vi "D2A_5V.vi"(0 "Channel to Cal":T2, 11 "Data In":dbl format="%0.2f", 13 "Cal Unit":T1) -> (15 "Data Out":dbl)   [LabVIEW 2019]
uses:
  Type Defs/New Channel Type Def (RIO).ctl
  Type Defs/Units Type Def (DAQ Rack).ctl
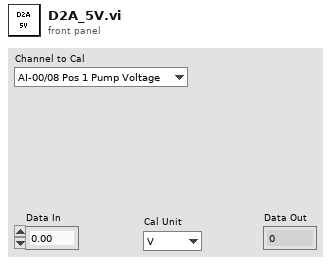
[diagram p1: front panel]
types:
  T1 = typedef "Units Type Def (DAQ Rack).ctl" = enum16{"V", "mA", "A", "Hz", "deg C"}
  T2 = typedef "New Channel Type Def (RIO).ctl" = enum16{"AI-00/08 Pos 1 Pump Voltage", "AI-01/09 Pos 2 Pump Voltage", "AI-02/10 Pos 3 Pump Voltage", "AI-03/11 Pos 4 Pump Voltage", "AI-04/12 Pos 5 Pump Voltage", "AI-05/13 Pos 6 Pump Voltage", "AI-06 Spare", "AI-14 Spare", "AI-07 Spare", "AI-15 Power Supply Voltage", "AI-16 Pos 1 Pump Current", "AI-17 Pos 2 Pump Current", "AI-18 Pos 3 Pump Current", "AI-19 Pos 4 Pump Current", "AI-20 Pos 5 Pump Current", "AI-21 Pos 6 Pump Current", "AI-16 Pos 1 Pump Speed", "AI-17 Pos 2 Pump Speed", "AI-18 Pos 3 Pump Speed", "AI-19 Pos 4 Pump Speed", "AI-20 Pos 5 Pump Speed", "AI-21 Pos 6 Pump Speed", "AI-22 Pos 1 Controller Current", "AI-23 Pos 2 Controller Current", "AI-24 Pos 3 Controller Current", "AI-25 Pos 4 Controller Current", "AI-26 Pos 5 Controller Current", "AI-27 Pos 6 Controller Current", "AI-28 Tank 1 Temperature", "AI-29 Tank 2 Temperature", "AI-30 Pos 1 Pump Pressure", "AI-31 Pos 2 Pump Pressure", "AI-32 Pos 3 Pump Pressure", "AI-33 Pos 4 Pump Pressure", "AI-34 Pos 5 Pump Pressure", "AI-35 Pos 6 Pump Pressure", "AI-36 Pos 1 Pump Flow", "AI-37 Pos 2 Pump Flow", "AI-38 Pos 3 Pump Flow", "AI-39 Pos 4 Pump Flow", "AI-40 Pos 5 Pump Flow", "AI-41 Pos 6 Pump Flow", "AI-42 Spare", "AI-43 Spare", "AI-44 Spare", "AI-45 Spare", "AI-46 Spare", "AI-47 Spare", "AI-00/08 Pos 1 Controller Voltage", "AI-01/09 Pos 2 Controller Voltage", "AI-02/10 Pos 3 Controller Voltage", "AI-03/11 Pos 4 Controller Voltage", "AI-04/12 Pos 5 Controller Voltage", "AI-05/13 Pos 6 Controller Voltage"}
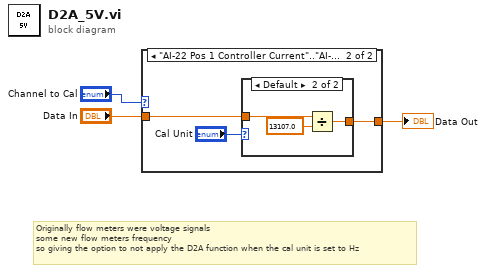
[diagram p0: block diagram]
diagram:
  # "Originally flow meters were voltage signals\nsome new flow meters frequency\nso giving the option to not apply the D2A function when the cal unit is set to Hz"
  n1 = case shown="\"AI-22 Pos 1 Controller Current\"..\"AI-47 Spare\"" "Channel to Cal" {
    tunnel: "Data In" -> [w4 w7]
    tunnel: [w4 w6] -> w1
    frame Default {
    }
    frame "AI-22 Pos 1 Controller Current".."AI-47 Spare" {
      n2 = case shown="Default" "Cal Unit" {
        tunnel: w7 -> [w8 w10]
        tunnel: [w8 w9] -> w6
        frame "Hz" {
        }
        frame Default {
          n3 = Divide(x=w10, y=13107.0) -> (x/y=w9:dbl)
        }
      }
    }
  }
  "Data Out" <- w1
